vi "Delete Macro.vi"(8 "error in (no error)":errorcluster, 10 "Delete Macro (\"\")":string, 11 "VISA resource name":refnum<visa-resource-name>) -> (0 "error out":errorcluster, 3 "VISA resource name out":refnum<visa-resource-name>)   [LabVIEW 2020, in "Rohde&Schwarz CMXP Base.lvlib"]
doc: "Deletes a macro.\n\nAttribute:\nRSCMXPBASE_ATTR_DELETE_MACRO\n\nRemote-control command:\n*RMC"
uses:
  <instrlib>/Rohde&Schwarz CMXP Base/Rohde&Schwarz CMXP Base.lvlib
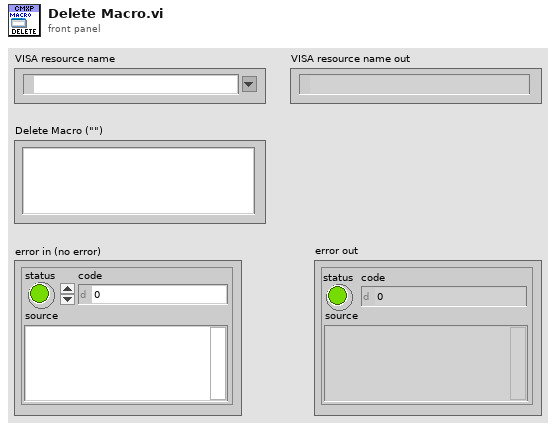
[diagram p1: front panel]
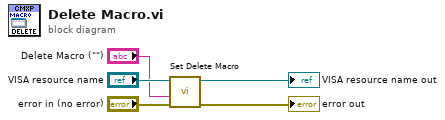
[diagram p0: block diagram]
diagram:
  n1 = call "Set Delete Macro"("error in (no error)"="error in (no error)", "Delete Macro ()"="Delete Macro (\"\")", "instrument handle"="VISA resource name") -> ("error out"=→"error out":errorcluster, "instrument handle out"=→"VISA resource name out":refnum<visa-resource-name>)  [unwired: 7 in]
